vi "MFLI_get_voltage -- V1.vi"(4 "Oscillator (0)":u16, 8 "Error In":errorcluster, 9 "timeconstant (s)":dbl=0.006, 10 "Freq IN (Hz)":dbl=40000.0 format="%#_13g", 11 "Handle In":T1 {"Handle" format="0x%08x"; "Conn" format="0x%08x"}) -> (0 "Error Out":errorcluster, 1 "z out (V)":cdb, 2 "Freq out (Hz)":dbl=40000.0 format="%#_13g", 3 "Handle Out":T1 {"Handle" format="0x%08x"; "Conn" format="0x%08x"})   [LabVIEW 2018]
uses:
  Applications/National Instruments/LabVIEW 2019 64-bit/instr.lib/Zurich Instruments LabOne/Zurich Instruments LabOne.lvlib
  Applications/National Instruments/LabVIEW 2019 64-bit/instr.lib/Zurich Instruments LabOne/Public/ziTypeHandle.ctl
panel:
  out "Phase OUT (deg)":dbl=40000.0 format="%#_13g"
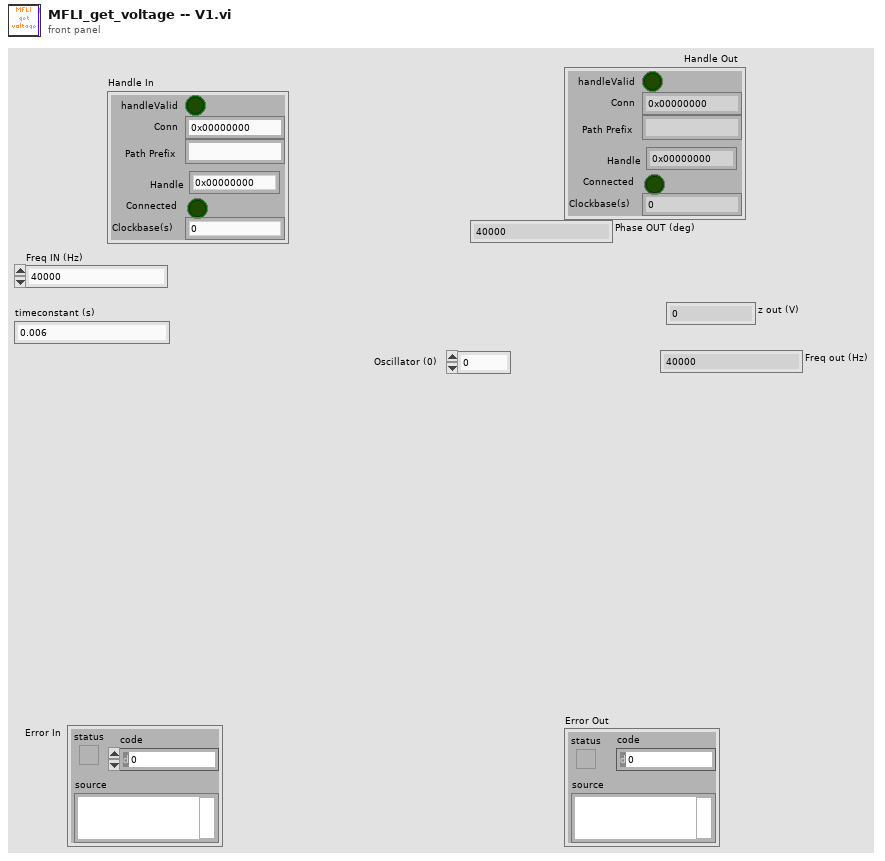
[diagram p1: front panel]
types:
  T1 = typedef "Zurich Instruments LabOne.lvlib/ziTypeHandle.ctl" = cluster{"handleValid":bool, "Conn":u64, "Path Prefix":string, "Handle":u64, "Connected":bool, "Clockbase(s)":dbl}
  T2 = typedef "Zurich Instruments LabOne.lvlib/ziTypeDemodSampleSingle.ctl" = cluster{"Timestamps (ticks)":u64, "X (Vrms)":dbl, "Y (Vrms)":dbl, "Osc Phase (deg)":dbl, "Freq (Hz)":dbl, "DIO":u32, "AuxIn0 (V)":dbl, "AuxIn1 (V)":dbl, "Trigger":u32}
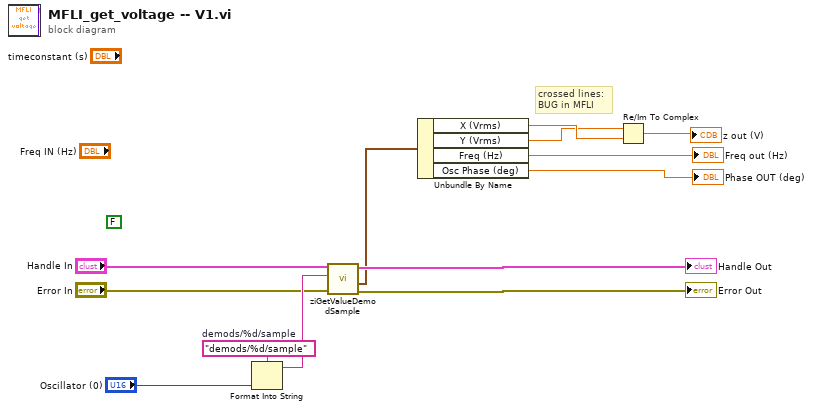
[diagram p0: block diagram]
diagram:
  (unwired) FALSE
  w10 = "demods/%d/sample"  # demods/%d/sample
  # "crossed lines:\nBUG in MFLI"
  n1 = Format Into String(format string=w10, "Oscillator (0)") -> (resulting string=w11:string)  [unwired: 2 in, 1 out]
  n2 = call "ziGetValueDemodSample.vi"("error in"="Error In", "Path"=w11, "Handle In"="Handle In") -> ("error out"=→"Error Out":errorcluster, "Demod Sample Out"=w9:T2, "Handle Out"=→"Handle Out":T1)  [unwired: 2 in]
  n3 = Unbundle By Name(w9) -> ("X (Vrms)"=w8:dbl, "Y (Vrms)"=w7:dbl, "Freq (Hz)"=→"Freq out (Hz)":dbl, "Osc Phase (deg)"=→"Phase OUT (deg)":dbl)
  n4 = Re/Im To Complex(1:w8, 2:w7) -> (0:→"z out (V)":cdb)
